vi "Parse Arguments.vi"(8 "error in (no error)":errorcluster, 10 "Inputs":string[](array[string]), 11 "LUnitCLI In":refnum<class "LUnitCLI.lvclass">) -> (0 "error out":errorcluster, 3 "LUnitCLI Out":refnum<class "LUnitCLI.lvclass">)   [LabVIEW 2020, in "LUnitCLI.lvclass"]
uses:
  LUnitCLI.lvclass
  LUnitCLI.lvclass/LUnitCLI.ctl
  <vilib>/ErrorRing/Error Ring.xnode
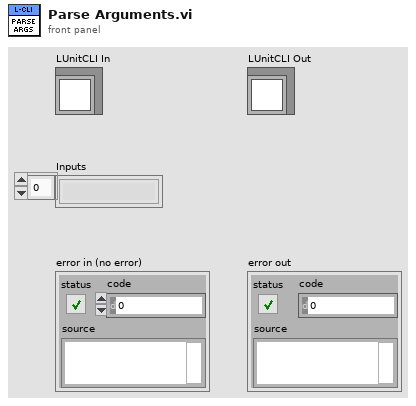
[diagram p1: front panel]
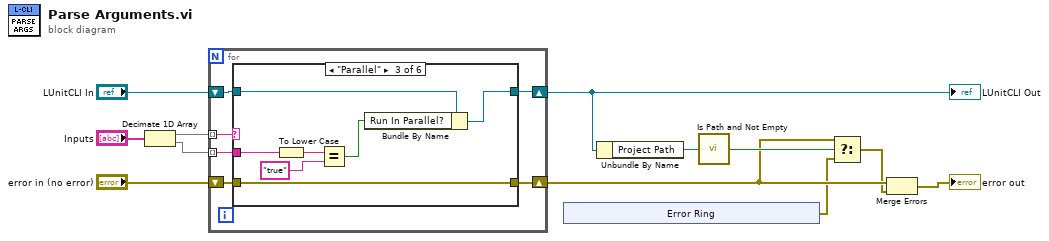
[diagram p0: block diagram]
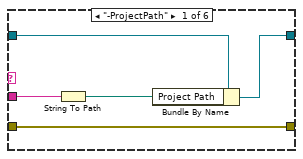
[diagram p2: hidden frame]
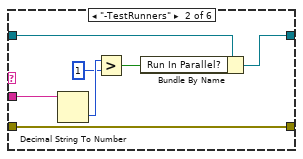
[diagram p3: hidden frame]
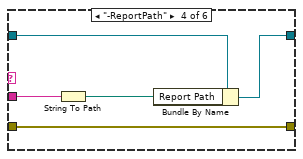
[diagram p4: hidden frame]
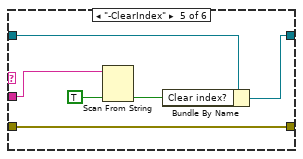
[diagram p5: hidden frame]
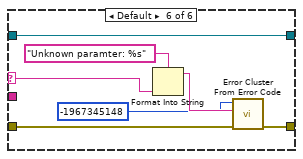
[diagram p6: hidden frame]
diagram:
  n1 = Decimate 1D Array("Inputs") -> (w9:string[], w10:string[])
  n2 = for {
    tunnel: w9 -> [w18] mode=indexing
    tunnel: w10 -> [w17] mode=indexing
    shift-right: [w15] -> w7
    shift-left: "LUnitCLI In" -> [w16]
    shift-right: [w14] -> w3
    shift-left: "error in (no error)" -> [w13]
    n3 = case shown="\"Parallel\"" w18 {
      selector: w18 -> [_ _ _ _ _ w54]
      tunnel: w17 -> [w20 w27 w34 w39 w45 _]
      tunnel: w16 -> [w23 w30 w37 w42 w48 w49]
      tunnel: [w22 w29 w36 w41 w47 w49] -> w15
      tunnel: [w21 w28 w35 w40 w46 w53] -> w14
      tunnel: w13 -> [w21 w28 w35 w40 w46 w50]
      frame "-ProjectPath" {
        n4 = String To Path(string=w20) -> (path=w19:path)
        n5 = Bundle By Name(cluster=w23, "Project Path"=w19) -> (w22:refnum<class "LUnitCLI.lvclass">)
      }
      frame "-TestRunners" {
        n6 = Decimal String To Number(string=w27) -> (number=w26:i32)  [unwired: 2 in, 1 out]
        n7 = Greater?(x=w26, y=1) -> (0:w24:bool)
        n8 = Bundle By Name(cluster=w30, "Run In Parallel?"=w24) -> (w29:refnum<class "LUnitCLI.lvclass">)
      }
      frame "Parallel" {
        n9 = To Lower Case(string=w34) -> (all lower case string=w33:string)
        n10 = Equal?(x=w33, y="true") -> (x = y?=w31:bool)
        n11 = Bundle By Name(cluster=w37, "Run In Parallel?"=w31) -> (w36:refnum<class "LUnitCLI.lvclass">)
      }
      frame "-ReportPath" {
        n12 = String To Path(string=w39) -> (path=w38:path)
        n13 = Bundle By Name(cluster=w42, "Report Path"=w38) -> (w41:refnum<class "LUnitCLI.lvclass">)
      }
      frame "-ClearIndex" {
        n14 = Scan From String(input string=w45, default 1=TRUE) -> (output 1=w44:bool)  [unwired: 3 in, 3 out]
        n15 = Bundle By Name(cluster=w48, "Clear index?"=w44) -> (w47:refnum<class "LUnitCLI.lvclass">)
      }
      frame Default {
        n16 = Format Into String(format string="Unknown paramter: %s", w54) -> (resulting string=w52:string)  [unwired: 2 in, 1 out]
        n17 = call <vilib>:"Error Cluster From Error Code.vi"("error in (no error)"=w50, "error message (\"\")"=w52, "error code (0)"=-1967345148) -> ("error out"=w53:errorcluster)  [unwired: 6 in]
      }
    }
  }
  "LUnitCLI Out" <- w7
  n18 = xnode "Error Ring"() -> ("error out"=w2:errorcluster)
  n19 = Unbundle By Name(w7) -> ("Project Path"=w6:path)
  n20 = call <vilib>:"Is Path and Not Empty.vi"("path"=w6) -> ("Is Path and Not Empty?"=w4:bool)  [unwired: 4 in]
  n21 = Select(t=w3, s=w4, f=w2) -> (s? t:f=w1:errorcluster)
  n22 = Merge Errors(w3, w1) -> (→"error out":errorcluster)
